vi "SysIdRoutine_Create.vi"(9 "Mechanism":T4, 11 "Config":T5={"m_timeout_Sec"=10.0, "m_stepVoltage_Volt"=7.0, "m_rampRate_V/S"=1.0}) -> (3 "SysIdRoutine":T3={"m_config"={"m_timeout_Sec"=10.0, "m_stepVoltage_Volt"=7.0, "m_rampRate_V/S"=1.0}, "m_mechanism"={"m_drive_volts"=0.0, "m_log"=[], "m_name"=""}, "m_outputVolts"=0.0, "m_recordState"=enum."kNone", "timer"={"StartTime"=0.0, "Accumulated TIme"=0.0, "Running"=FALSE, "semaphore"=refnum}} {"timer"."Accumulated TIme" format="%13.5p"; "timer"."StartTime" format="%13.5p"})   [LabVIEW 2023]
uses:
  <vilib>/Rock Robotics/WPI/ThirdParty/JAS_Junk/TrajLib/TypeDef/TIMER.ctl
  impl_ControlRecordType_ENUM.ctl
  <vilib>/Rock Robotics/WPI/ThirdParty/JAS_Junk/TrajLib/Trajectory_Library.lvlib
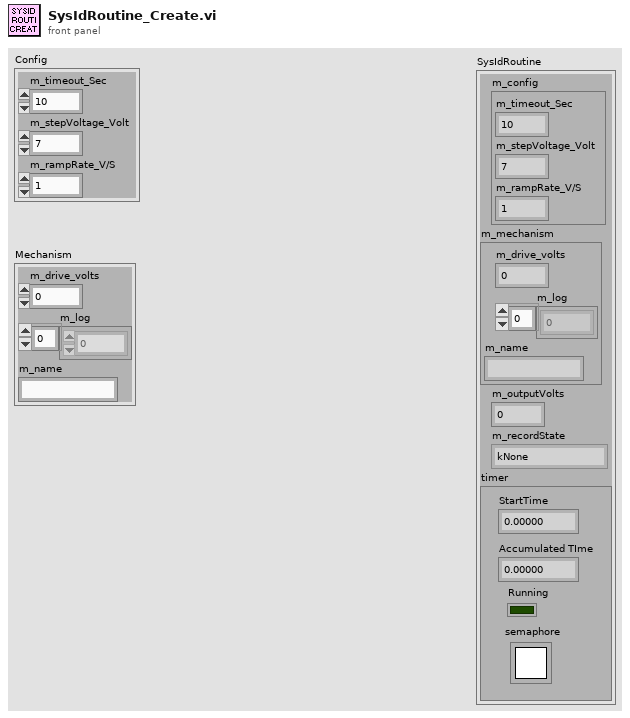
[diagram p1: front panel]
types:
  T1 = typedef "Trajectory_Library.lvlib/TIMER.ctl" = cluster{"StartTime":dbl, "Accumulated TIme":dbl, "Running":bool, "semaphore":T2}
  T2 = typedef "Semaphore RefNum" = refnum<k1>
  T3 = cluster{"m_config":cluster{"m_timeout_Sec":dbl, "m_stepVoltage_Volt":dbl, "m_rampRate_V/S":dbl}, "m_mechanism":cluster{"m_drive_volts":dbl, "m_log":u8[], "m_name":string}, "m_outputVolts":dbl, "m_recordState":enum16{"kQuasistaticForward", "kQuasistaticReverse", "kDynamicForward", "kDynamicReverse", "kNone"}, "timer":T1}
  T4 = cluster{"m_drive_volts":dbl, "m_log":u8[], "m_name":string}
  T5 = cluster{"m_timeout_Sec":dbl, "m_stepVoltage_Volt":dbl, "m_rampRate_V/S":dbl}
  T6 = typedef "impl_ControlRecordType_ENUM.ctl" = enum16{"kControlStart", "kControlFinish", "kControlSetMetadata"}
  T7 = cluster{"entry ID being started/completed/updated":i32, "entry name UTF-8 string data (arbitrary length)":string, "entry type UTF-8 string data (arbitrary length)":string, "entry metadata UTF-8 string data (arbitrary length)":string}
  T8 = enum16{"kQuasistaticForward", "kQuasistaticReverse", "kDynamicForward", "kDynamicReverse"}[]
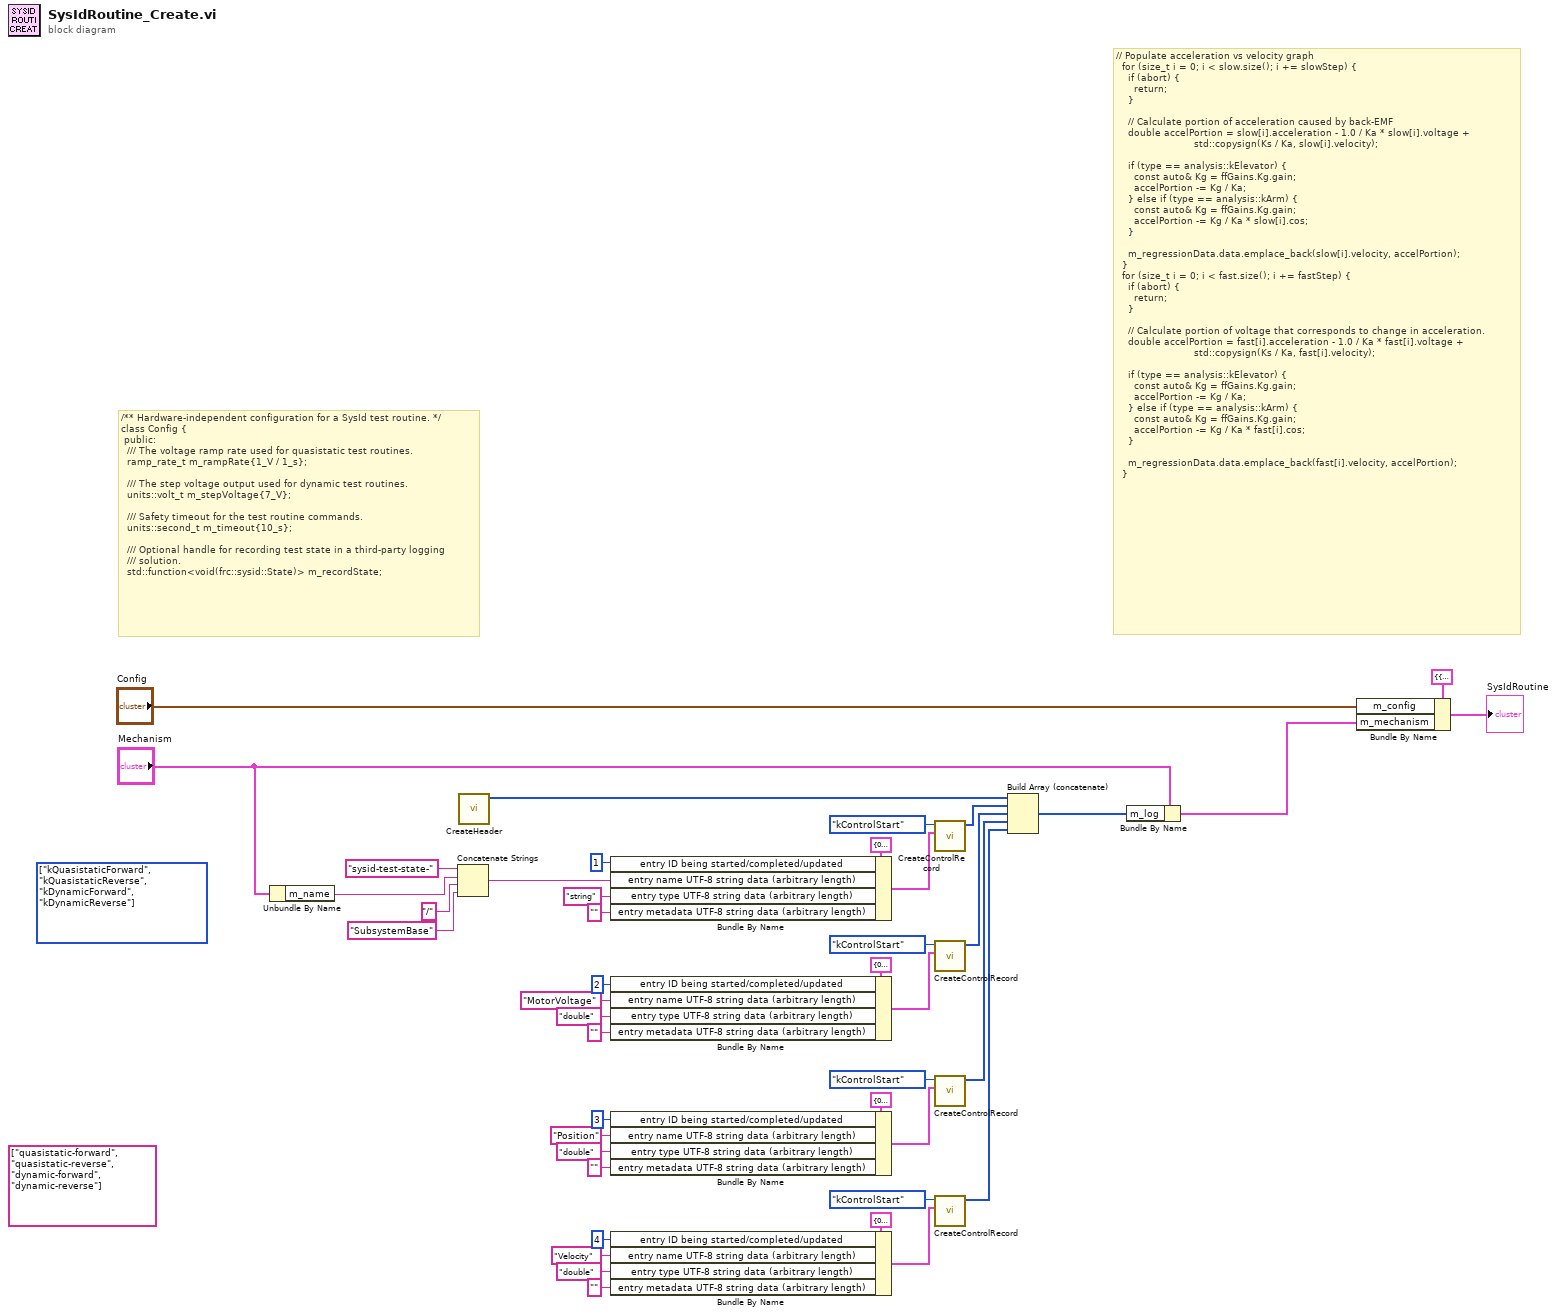
[diagram p0: block diagram]
diagram:
  (unwired) string[] ["quasistatic-forward", "quasistatic-reverse", "dynamic-forward", "dynamic-reverse"]
  (unwired) T8 [enum."kQuasistaticForward", enum."kQuasistaticReverse", enum."kDynamicForward", enum."kDynamicReverse"] items=["kQuasistaticForward", "kQuasistaticReverse", "kDynamicForward", "kDynamicReverse"]
  # "/** Hardware-independent configuration for a SysId test routine. */\nclass Config {\n public:\n  /// The voltage ramp rate used for quasistatic test routines.\n  ramp_rate_t m_rampRate{1_V / 1_s};\n\n  /// The step voltage output used for dynamic test routines.\n  units::volt_t m_stepVoltage{7_V};\n\n  /// Safety timeout for the test routine commands.\n  units::second_t m_timeout{10_s};\n\n  /// Optional handle for recording test state in a third-party logging\n  /// solution.\n  std::function<void(frc::sysid::State)> m_recordState;"
  # "// Populate acceleration vs velocity graph\n  for (size_t i = 0; i < slow.size(); i += slowStep) {\n    if (abort) {\n      return;\n    }\n\n    // Calculate portion of acceleration caused by back-EMF\n    double accelPortion = slow[i].acceleration - 1.0 / Ka * slow[i].voltage +\n                          std::copysign(Ks / Ka, slow[i].velocity);\n\n    if (type == analysis::kElevator) {\n      const auto& Kg = ffGains.Kg.gain;\n      accelPortion -= Kg / Ka;\n    } else if (type == analysis::kArm) {\n      const auto& Kg = ffGains.Kg.gain;\n      accelPortion -= Kg / Ka * slow[i].cos;\n    }\n\n    m_regressionData.data.emplace_back(slow[i].velocity, accelPortion);\n  }\n  for (size_t i = 0; i < fast.size(); i += fastStep) {\n    if (abort) {\n      return;\n    }\n\n    // Calculate portion of voltage that corresponds to change in acceleration.\n    double accelPortion = fast[i].acceleration - 1.0 / Ka * fast[i].voltage +\n                          std::copysign(Ks / Ka, fast[i].velocity);\n\n    if (type == analysis::kElevator) {\n      const auto& Kg = ffGains.Kg.gain;\n      accelPortion -= Kg / Ka;\n    } else if (type == analysis::kArm) {\n      const auto& Kg = ffGains.Kg.gain;\n      accelPortion -= Kg / Ka * fast[i].cos;\n    }\n\n    m_regressionData.data.emplace_back(fast[i].velocity, accelPortion);\n  }"
  n1 = Unbundle By Name("Mechanism") -> ("m_name"=w1:string)
  n2 = Concatenate Strings("sysid-test-state-" ("string"), w1, "/" ("string"), "SubsystemBase" ("entry name UTF-8 string data (arbitrary length)")) -> (w8:string)
  n3 = call "CreateHeader.vi"() -> ("header"=w17:u8[])  [unwired: 11 in]
  n4 = Bundle By Name(cluster=T7 {"entry ID being started/completed/updated"=0, "entry name UTF-8 string data (arbitrary length)"="", "entry type UTF-8 string data (arbitrary length)"="", "entry metadata UTF-8 string data (arbitrary length)"=""} ("Control Record Payload Data"), "entry ID being started/completed/updated"=1, "entry name UTF-8 string data (arbitrary length)"=w8, "entry type UTF-8 string data (arbitrary length)"="string", "entry metadata UTF-8 string data (arbitrary length)"="") -> (w36:T7)
  n5 = Bundle By Name(cluster=T7 {"entry ID being started/completed/updated"=0, "entry name UTF-8 string data (arbitrary length)"="", "entry type UTF-8 string data (arbitrary length)"="", "entry metadata UTF-8 string data (arbitrary length)"=""} ("Control Record Payload Data"), "entry ID being started/completed/updated"=2, "entry name UTF-8 string data (arbitrary length)"="MotorVoltage", "entry type UTF-8 string data (arbitrary length)"="double", "entry metadata UTF-8 string data (arbitrary length)"="") -> (w37:T7)
  n6 = Bundle By Name(cluster=T7 {"entry ID being started/completed/updated"=0, "entry name UTF-8 string data (arbitrary length)"="", "entry type UTF-8 string data (arbitrary length)"="", "entry metadata UTF-8 string data (arbitrary length)"=""} ("Control Record Payload Data"), "entry ID being started/completed/updated"=3, "entry name UTF-8 string data (arbitrary length)"="Position", "entry type UTF-8 string data (arbitrary length)"="double", "entry metadata UTF-8 string data (arbitrary length)"="") -> (w39:T7)
  n7 = Bundle By Name(cluster=T7 {"entry ID being started/completed/updated"=0, "entry name UTF-8 string data (arbitrary length)"="", "entry type UTF-8 string data (arbitrary length)"="", "entry metadata UTF-8 string data (arbitrary length)"=""} ("Control Record Payload Data"), "entry ID being started/completed/updated"=4, "entry name UTF-8 string data (arbitrary length)"="Velocity", "entry type UTF-8 string data (arbitrary length)"="double", "entry metadata UTF-8 string data (arbitrary length)"="") -> (w38:T7)
  n8 = call "CreateControlRecord.vi"("Control Record Payload Data"=w36, "ControlRecordType"=impl_ControlRecordType_ENUM."kControlStart") -> ("control record"=w40:u8[])  [unwired: 9 in]
  n9 = call "CreateControlRecord.vi"("Control Record Payload Data"=w37, "ControlRecordType"=impl_ControlRecordType_ENUM."kControlStart") -> ("control record"=w41:u8[])  [unwired: 9 in]
  n10 = call "CreateControlRecord.vi"("Control Record Payload Data"=w39, "ControlRecordType"=impl_ControlRecordType_ENUM."kControlStart") -> ("control record"=w42:u8[])  [unwired: 9 in]
  n11 = call "CreateControlRecord.vi"("Control Record Payload Data"=w38, "ControlRecordType"=impl_ControlRecordType_ENUM."kControlStart") -> ("control record"=w43:u8[])  [unwired: 9 in]
  n12 = Build Array (concatenate)(w17, w40, w41, w42, w43) -> (w7:u8[])
  n13 = Bundle By Name(cluster="Mechanism", "m_log"=w7) -> (w4:T4)
  n14 = Bundle By Name(cluster=T3 {"m_config"={"m_timeout_Sec"=10.0, "m_stepVoltage_Volt"=7.0, "m_rampRate_V/S"=1.0}, "m_mechanism"={"m_drive_volts"=0.0, "m_log"=[], "m_name"=""}, "m_outputVolts"=0.0, "m_recordState"=enum."kNone", "timer"={"StartTime"=0.0, "Accumulated TIme"=0.0, "Running"=FALSE, "semaphore"=refnum}} ("SysIdRoutine"), "m_config"="Config", "m_mechanism"=w4) -> (→"SysIdRoutine":T3)
